vi "JSONExample.vi"() -> ()   [LabVIEW 2017]
panel:
  in  "port":u16=5557
  in  "Stop Button":bool
  out "time (ms)":dbl
  out "split name":string[](array[string])
  out "name":string
  out "thresholds":sgl[](array[numeric]) format="%.2f"
  out "sample rate":sgl format="%.2f"
  out "timestamp":i64
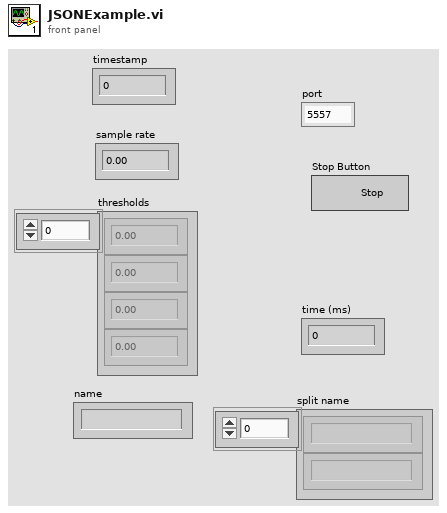
[diagram p1: front panel]
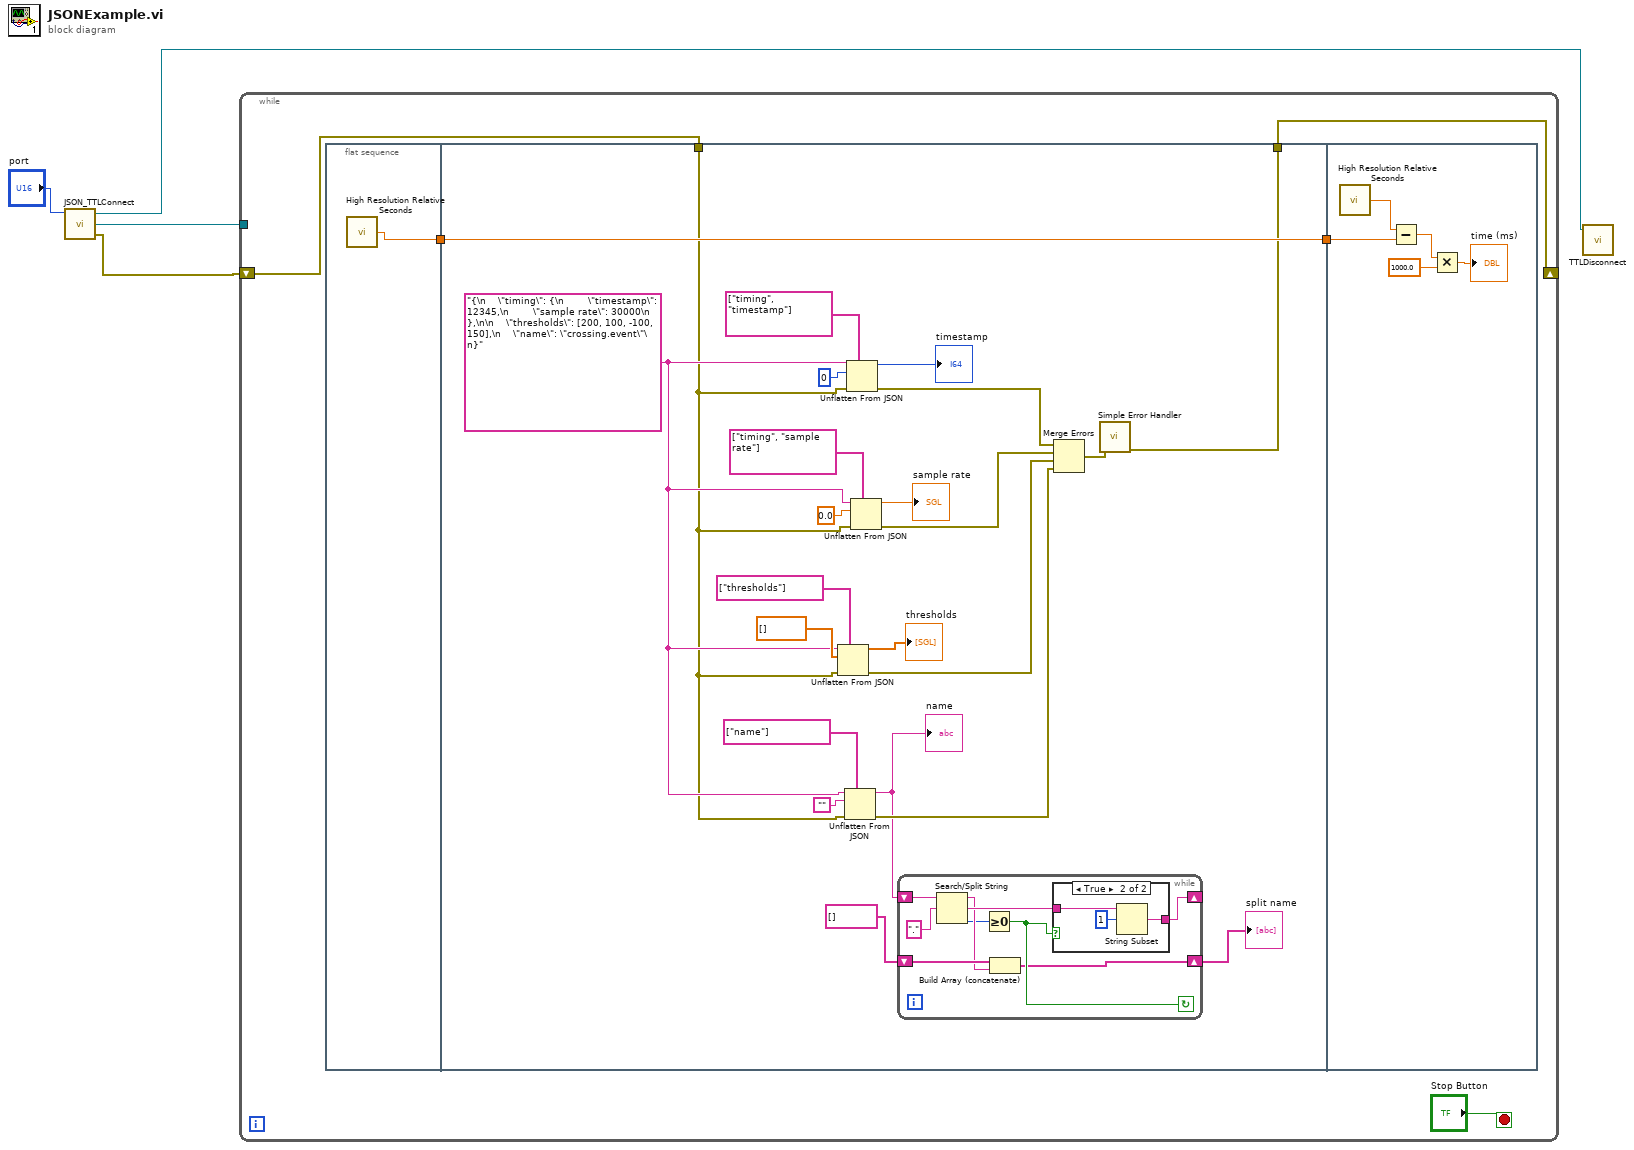
[diagram p0: block diagram]
diagram:
  n1 = call "JSON_TTLConnect.vi"("port"="port") -> ("context out"=w4:refnum<class "zmq_context.lvclass">, "socket out"=w1:refnum<class "zmq_socket.lvclass">, "error out"=w2:errorcluster)  [unwired: 4 in]
  n2 = while {
    shift-right: [w5] -> _
    shift-left: w2 -> [w6]
    tunnel: w1 -> [_]
    stop <- "Stop Button" stop-if-true
    n3 = flat-sequence {
      tunnel: [w10] -> w9
      tunnel: w9 -> [w15]
      tunnel: [w15] -> w8
      tunnel: w6 -> [w11]
      tunnel: [w12] -> w5
      tunnel: w8 -> [w50]
      frame #0 {
        n4 = call <vilib>:"High Resolution Relative Seconds.vi"() -> ("relative seconds"=w10:dbl)
      }
      frame #1 {
        w18 = "{\n    \"timing\": {\n        \"timestamp\": 12345,\n        \"sample rate\": 30000\n    },\n\n    \"thresholds\": [200, 100, -100, 150],\n    \"name\": \"crossing.event\"\n}"
        n5 = Unflatten From JSON(path=string[] ["thresholds"], JSON string=w18, type and defaults=sgl[] [], error in (no error)=w11) -> (value=→"thresholds":sgl[], error out=w21:errorcluster)  [unwired: 3 in]
        n6 = Unflatten From JSON(path=string[] ["name"], JSON string=w18, type and defaults="", error in (no error)=w11) -> (value=w16:string, error out=w17:errorcluster)  [unwired: 3 in]
        "name" <- w16
        n7 = Unflatten From JSON(path=string[] ["timing", "timestamp"], JSON string=w18, type and defaults=i64 0, error in (no error)=w11) -> (value=→"timestamp":i64, error out=w30:errorcluster)  [unwired: 3 in]
        n8 = Unflatten From JSON(path=string[] ["timing", "sample rate"], JSON string=w18, type and defaults=sgl 0.0, error in (no error)=w11) -> (value=→"sample rate":sgl, error out=w25:errorcluster)  [unwired: 3 in]
        n9 = while {
          shift-right: [w41] -> _
          shift-left: w16 -> [w42]
          shift-right: [w35] -> w13
          shift-left: string[] [] ("Array") -> [w39]
          stop <- w36 continue-if-true
          n10 = Search/Split String(string=w42, search string/char (-)=".") -> (substring before match=w38:string, match + rest of string=w40:string, offset of match=w37:i32)  [unwired: 1 in]
          n11 = Greater Or Equal To 0?(x=w37) -> (x >= 0?=w36:bool)
          n12 = Build Array (concatenate)(w39, w38) -> (w35:string[])
          n13 = case shown="True" w36 {
            tunnel: [w43 w46] -> w41
            tunnel: w40 -> [w43 w45]
            frame False {
            }
            frame True {
              n14 = String Subset(string=w45, offset (0)=1) -> (substring=w46:string)  [unwired: 1 in]
            }
          }
        }
        "split name" <- w13
        n15 = Merge Errors(w30, w25, w21, w17) -> (w31:errorcluster)
        n16 = call <vilib>:"Simple Error Handler.vi"("error in (no error)"=w31) -> ("error out"=w12:errorcluster)  [unwired: 4 in, 4 out]
      }
      frame #2 {
        n17 = call <vilib>:"High Resolution Relative Seconds.vi"() -> ("relative seconds"=w51:dbl)
        n18 = Subtract(x=w51, y=w50) -> (x-y=w49:dbl)
        n19 = Multiply(x=w49, y=1000.0) -> (x*y=→"time (ms)":dbl)
      }
    }
  }
  n20 = call "TTLDisconnect.vi"("context in"=w4) -> ()  [unwired: 3 in, 1 out]
